vi "BartlomiejLechman_prac9_1.vi"   [LabVIEW 2019]
uses:
  <vilib>/Platform/TimedLoop/XDataNode/timing_clust.ctl
  <vilib>/Platform/TimedLoop/XDataNode/nitl_modes.ctl
  <vilib>/Platform/TimedLoop/XDataNode/wakeup.ctl
  <vilib>/platform/TimedLoop/XDataNode/XDataNode.xnode
  <vilib>/Platform/TimedLoop/XDataNode/XDNodeRunTimeDep.lvlib
  <vilib>/measure/NI_MABase.lvlib
types:
  T1 = typedef "XDNodeRunTimeDep.lvlib/timing_clust.ctl" = cluster{"Expected End [f-1]":u64, "Actual End [f-1]":u64, "Finished Late? [f-1]":bool, "Expected End [i-1]":u64, "Actual End [i-1]":u64, "Finished Late? [i-1]":bool, "Expected Start [i]":u64, "Actual Start [i]":u64, "Expected Start [f]":u64, "Actual Start [f]":u64, "Source Name":string, "Structure Name":string, "Period":i64, "Deadline":i64, "Offset":i64, "Start":i64, "Priority":i32, "Timeout":i32, "Mode":T2, "Wakeup Reason":T3, "Error":errorcluster, "Source Type":string, "Secondary Source Type":string, "Global End Time":u64, "Global Start Time":u64, "Frame Duration":u64, "Iteration Duration":u64, "Assigned CPU":i32, "I/O Scan Engine Mode":u32}
  T2 = typedef "XDNodeRunTimeDep.lvlib/nitl_modes.ctl" = enum32{"No Change", "Process missed periods, maintain original phase", "Discard missed periods, maintain original phase", "Process missed periods, ignore original phase", "Discard missed periods, ignore original phase"}
  T3 = typedef "XDNodeRunTimeDep.lvlib/wakeup.ctl" = enum32{"Normal", "Aborted", "Asynchronous wakeup", "Timing source error", "Timed loop error", "Timeout"}
  T4 = enum16{"Sine Wave", "Triangle Wave", "Square Wave", "Sawtooth Wave"}
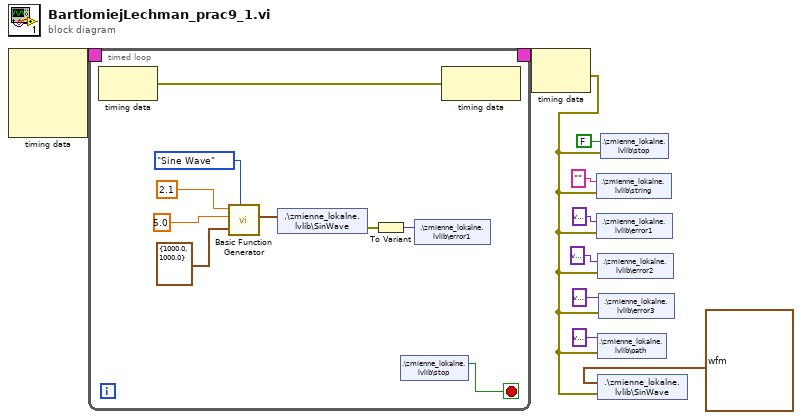
[diagram p0: block diagram]
diagram:
  n1 = node-c288() -> (w10:T1)  [unwired: 4 in]
  n2 = timed-loop {
    timing: w10 -> [_]
    timing-out: [_] -> w9
    stop <- w14 stop-if-true
    n3 = node-c288() -> (w11:errorcluster)  [unwired: 1 in]
    n4 = call <vilib>:"Basic Function Generator.vi"("sampling info"=cluster{"Fs":dbl, "#s":dbl} {"Fs"=1000.0, "#s"=1000.0}, "signal type"=T4."Sine Wave", "amplitude"=5.0, "frequency"=2.1) -> ("signal out"=w15:waveform(dbl))  [unwired: 5 in, 2 out]
    n5 = shared-variable ".\\zmienne_lokalne.lvlib\\SinWave"(w15) -> (error out=w12:errorcluster)  [unwired: 1 in]
    n6 = To Variant(anything=w12) -> (Variant=w13:variant)
    n7 = shared-variable ".\\zmienne_lokalne.lvlib\\stop"() -> (w14:bool)  [unwired: 1 in, 1 out]
    n8 = shared-variable ".\\zmienne_lokalne.lvlib\\error1"(w13) -> ()  [unwired: 1 in, 1 out]
    n9 = node-c288(w11) -> ()  [unwired: 1 out]
  }
  n10 = node-c288(w9) -> (w6:errorcluster)
  n11 = shared-variable ".\\zmienne_lokalne.lvlib\\string"("" ("napis"), error in=w6) -> ()  [unwired: 1 out]
  n12 = shared-variable ".\\zmienne_lokalne.lvlib\\error1"(variant ("error1"), error in=w6) -> ()  [unwired: 1 out]
  n13 = shared-variable ".\\zmienne_lokalne.lvlib\\error2"(variant ("error2"), error in=w6) -> ()  [unwired: 1 out]
  n14 = shared-variable ".\\zmienne_lokalne.lvlib\\path"(variant ("path"), error in=w6) -> ()  [unwired: 1 out]
  n15 = shared-variable ".\\zmienne_lokalne.lvlib\\SinWave"(waveform(dbl) {"t0"=timestamp(0 s since 1904-01-01), "dt"=1.0, "Y"=[]} ("SinWave"), error in=w6) -> ()  [unwired: 1 out]
  n16 = shared-variable ".\\zmienne_lokalne.lvlib\\error3"(variant ("error3"), error in=w6) -> ()  [unwired: 1 out]
  n17 = shared-variable ".\\zmienne_lokalne.lvlib\\stop"(FALSE ("stop"), error in=w6) -> ()  [unwired: 1 out]
